vi "Change Input Tag.vi"(6 "Variant":variant, 8 "error in (no error)":errorcluster, 9 "old values":string[][](array[string]), 10 "object ref in":T1, 11 "Cluster":T2) -> (0 "error out":errorcluster)   [LabVIEW 2013, in "Scaling editor node.lvclass"]
uses:
  Scaling editor node.lvclass
  <vilib>/NI/DCAF/Tag Editor Core/Table API/Table Manager/Cell Change.ctl
  <vilib>/NI/DCAF/Tag Editor Core/Table API/Table Manager/object ref.ctl
  <vilib>/NI/DCAF/Tag Editor Core/Configuration Editor/Classes/Engine Parent/Engine Parent Editor Node.lvclass
  <vilib>/NI/DCAF/Tag Editor Core/Configuration Editor/Classes/Module editor node/module editor node.lvclass
  <vilib>/NI/Tag Bus Module Framework/channel/TBM channel.lvclass
  module/configuration/Scaling configuration.lvclass
  Scaling editor node.lvclass/Scaling editor node.ctl
  <vilib>/NI/DCAF/Tag Editor Core/Table API/Table Manager.lvlib
  <vilib>/NI/DCAF/Tag Editor Core/Table API/Table Manager/Table Manager.lvclass
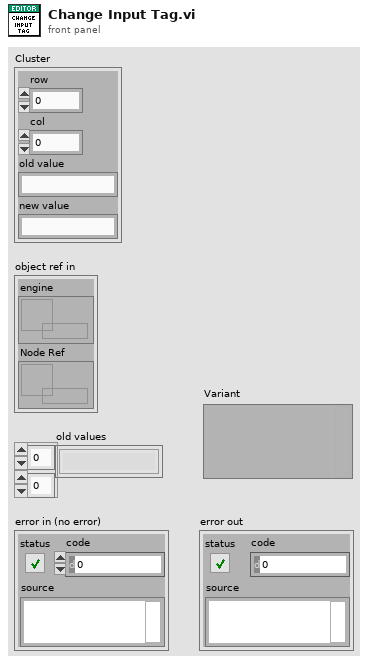
[diagram p1: front panel]
types:
  T1 = typedef "Table Manager.lvlib/Table Manager.lvclass/object ref.ctl" = cluster{"engine":refnum<data-value>, "Node Ref":refnum<data-value>}
  T2 = typedef "Table Manager.lvlib/Cell Change.ctl" = cluster{"row":i32, "col":i32, "old value":string, "new value":string}
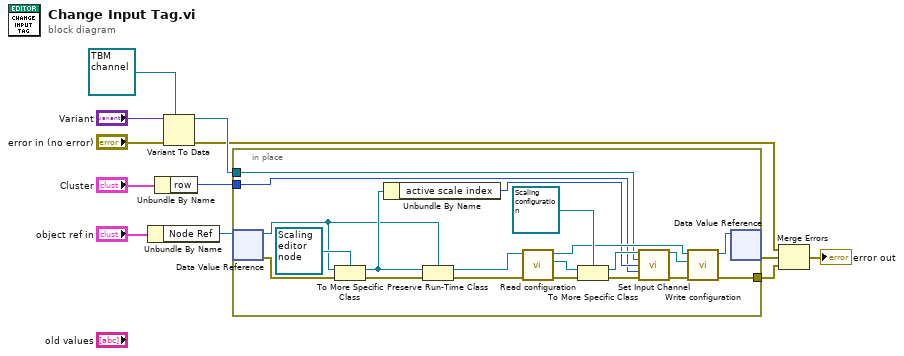
[diagram p0: block diagram]
diagram:
  n1 = Unbundle By Name("object ref in") -> ("Node Ref"=w11:refnum<data-value>)
  n2 = Unbundle By Name("Cluster") -> ("row"=w6:i32)
  n3 = Variant To Data(error in="error in (no error)", type=refnum<class "TBM channel.lvclass"> refnum ("output"), Variant="Variant") -> (data=w8:refnum<class "TBM channel.lvclass">, error out=w2:errorcluster)
  n4 = in-place {
    in-place-border: w8 -> [w18]
    in-place-border: w6 -> [w16]
    in-place-border: [w19] -> w3
    n5 = in-place-dvr #1(w11) -> (w15:refnum<class "module editor node.lvclass">, w14:errorcluster)
    n6 = To More Specific Class(target class=refnum<class "Scaling editor node.lvclass"> refnum ("Scaling editor node"), reference=w15, error in=w14) -> (specific class reference=w28:refnum<class "Scaling editor node.lvclass">, error out=w13:errorcluster)
    n7 = Unbundle By Name(w28) -> ("active scale index"=w17:i32)
    n8 = Preserve Run-Time Class(object in=w28, error in=w13, 2:w15) -> (object out=w27:refnum<class "module editor node.lvclass">, error out=w26:errorcluster)
    n9 = call-dynamic "Read configuration.vi"("error in"=w26, "NISE_CEF_serializable node in"=w27) -> ("error out"=w24:errorcluster, "configuration"=w30:refnum<class "NISE_CEF_serializable configuration.lvclass">, "NISE_CEF_serializable node out"=w21:refnum<class "module editor node.lvclass">)  [unwired: 7 in]
    n10 = To More Specific Class(target class=refnum<class "Scaling configuration.lvclass"> refnum ("Scaling configuration"), reference=w30, error in=w24) -> (specific class reference=w23:refnum<class "Scaling configuration.lvclass">, error out=w25:errorcluster)
    n11 = call "Set Input Channel.vi"("Scaling configuration in"=w23, "Channel"=w18, "Scale Index"=w17, "Mapping Index"=w16, "error in (no error)"=w25) -> ("Scaling configuration out"=w22:refnum<class "Scaling configuration.lvclass">, "error out"=w20:errorcluster)  [unwired: 9 in]
    n12 = call-dynamic "Write configuration.vi"("error in"=w20, "configuration"=w22, "NISE_CEF_serializable node in"=w21) -> ("error out"=w19:errorcluster, "NISE_CEF_serializable node out"=w32:refnum<class "module editor node.lvclass">)  [unwired: 7 in]
    n13 = in-place-dvr #1(w32) -> (w4:errorcluster)  [unwired: 1 out]
  }
  n14 = Merge Errors(w2, w4, w3) -> (→"error out":errorcluster)
